vi "Read Camera Controller Auto Redraw.vi"(8 "error in (no error)":errorcluster, 11 "SceneGraphDisplay.lvclass in":refnum<class "SceneGraphDisplay.lvclass">) -> (0 "error out":errorcluster, 2 "CameraController.AutoRedraw":bool, 3 "SceneGraphDisplay.lvclass out":refnum<class "SceneGraphDisplay.lvclass">)   [LabVIEW 2015, in "SceneGraphDisplay.lvclass"]
uses:
  SceneGraphDisplay.lvclass
  SceneGraphDisplay.lvclass/SceneGraphDisplay.ctl
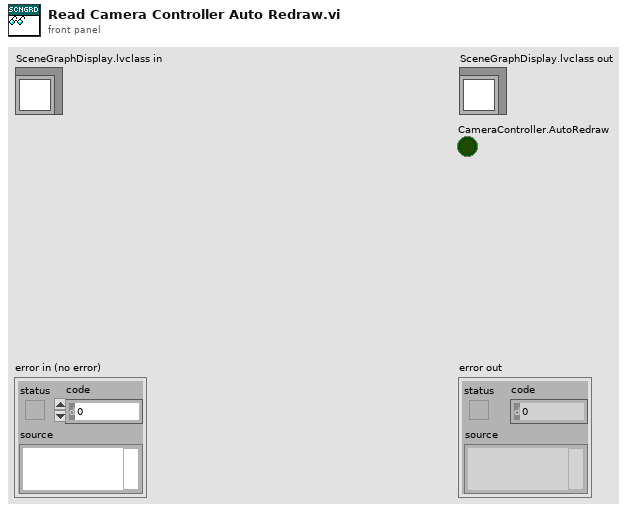
[diagram p1: front panel]
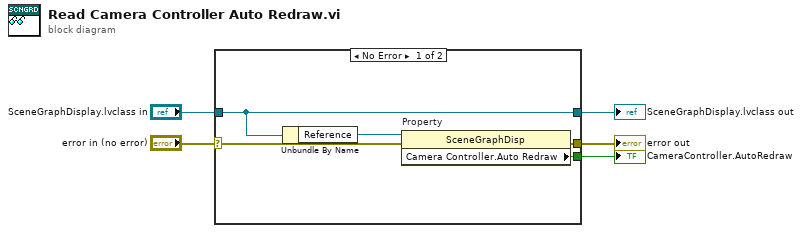
[diagram p0: block diagram]
diagram:
  n1 = case shown="No Error" "error in (no error)" {
    selector: "error in (no error)" -> [w6 w12]
    tunnel: [w9 w12] -> w4
    tunnel: [w8 w11] -> w2
    tunnel: "SceneGraphDisplay.lvclass in" -> [w8 w11]
    tunnel: [w10 _] -> w1
    frame No Error {
      n2 = Unbundle By Name(w8) -> ("Reference"=w7:refnum<vi>)
      n3 = property on="Property" class="SceneGraphDisp"(reference=w7, error in=w6) -> (error out=w9:errorcluster, "Camera Controller.Auto Redraw"=w10:bool)  [unwired: 1 out]
    }
    frame Error {
    }
  }
  "error out" <- w4
  "SceneGraphDisplay.lvclass out" <- w2
  "CameraController.AutoRedraw" <- w1
